vi "Get 8 Neighbors.vi"(9 "Column":i32, 10 "Row":i32, 11 "cells in":T1) -> (3 "cells living":bool[](array[boolean]))   [LabVIEW 2020, in "Game Of Life.lvlib"]
uses:
  Game Of Life.lvlib
  Game Board.ctl
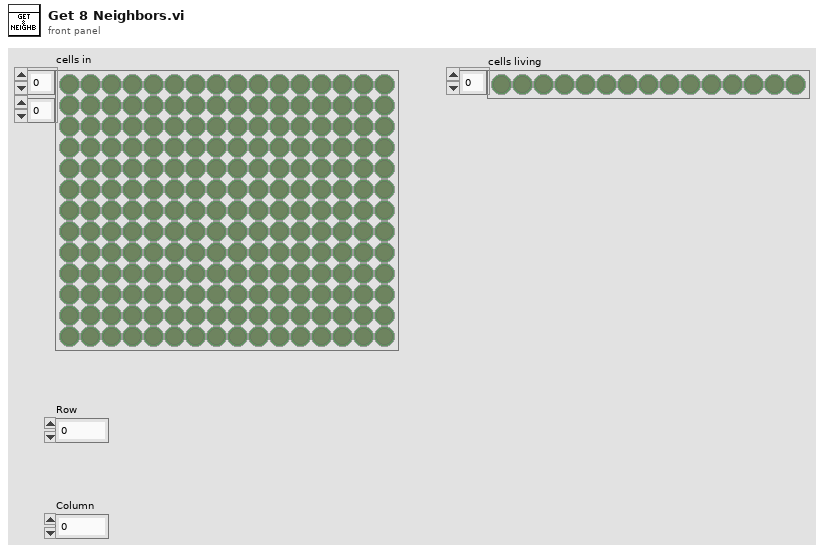
[diagram p1: front panel]
types:
  T1 = typedef "Game Of Life.lvlib/Game Board.ctl" = bool[][]
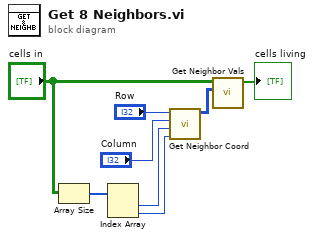
[diagram p0: block diagram]
diagram:
  n1 = Array Size(array="cells in") -> (size(s)=w8:i32[])
  n2 = Index Array(array=w8) -> (element #1=w5:i32, element #2=w4:i32)  [unwired: 2 in]
  n3 = call "Get Neighbor Coord.vi"("# cols"=w4, "# rows"=w5, "Column"="Column", "Row"="Row") -> ("Neighbor Coordinates"=w2:i32[][])  [unwired: 7 in]
  n4 = call "Get Neighbor Vals.vi"("Neighbor Coordinates"=w2, "cells in"="cells in") -> ("cells living"=→"cells living":bool[])  [unwired: 9 in]
